vi "Initialize.vi"(8 "ErrorIn":errorcluster, 10 "Modul Type to Simulate":T1 items=["Hardware Modus"=0, "SPC-600 Simulation"=600, "SPC-630 Simulation"=630, "SPC-700  Simulation"=700, "SPC-730  Simulation"=730, "SPC-130  Simulation"=130, "SPC-830  Simulation"=830, "SPC-140  Simulation"=140, "SPC-930  Simulation"=930, "DPC-230  Simulation"=230, "SPC-150  Simulation"=150, "SPC-150 N  Simulation"=151, "SPC-150 NX  Simulation"=152, "SPC-130 EM  Simulation"=131, "SPC-130 EMN  Simulation"=132, "SPC-130 IN Simulation"=135, "SPC-130 INX Simulation"=136, "SPC-130 INXX Simulation"=137, "SPC-160  Simulation"=160, "SPC-160 X  Simulation"=161, "SPC-160 PCIE  Simulation"=162, "SPC-180 Simulation"=180, "SPC-181 Simulation"=181, "SPC-182 Simulation"=182, "SPC-185 Simulation"=185, "SPC-186 Simulation"=186, "SPC-187 Simulation"=187, "DPC-330  Simulation"=330, "DPC-590  Simulation"=590, "TDC-104 Simulation"=104, "TDC-004 Simulation"=4, "TDC-106 Simulation"=106]) -> (0 "ErrorOut":errorcluster, 1 "SerialNumbersArray":string[](array[string]), 2 "ModuleNoArray":i16[](array[numeric]), 3 "DLL Path":path, 5 "SPCModulesArray":T2[](array[typedef]) {"Bus Number" min=-1 max=255 step=1; "Base I/O Addr" format="%.0x"; "Init Status" min=-10 max=0 step=1; "in Use" min=-1 max=1 step=1; "Slot Number" min=-1 max=255 step=1; "Module Type" items=["SPC-600"=600, "SPC-630"=630, "SPC-700"=700, "SPC-730"=730, "SPC-130"=130, "SPC-830"=830, "SPC-140"=140, "SPC-930"=930, "DPC-230"=230, "SPC-150"=150, "SPC-150 N"=151, "SPC-150 NX"=152, "SPC-130 EM"=131, "SPC-130 EMN"=132, "SPC-130IN"=135, "SPC-130INX"=136, "SPC-130INXX"=137, "SPC-160"=160, "SPC-160 X"=161, "SPC-160 PCIE"=162, "SPC-180 N"=180, "SPC-180 NX"=181, "SPC-180 NXX"=182, "SPC-180 N-USB"=185, "SPC-180 NX-USB"=186, "SPC-180 NXX-USB"=187, "SPC-QC-104"=104, "SPC-QC-004"=4, "SPC-QC-106"=106, "DPC-330"=330, "PMS-800"=800, "SPC-590"=590, "Simulation"=-1]})   [LabVIEW 2023]
doc: "This is a convenience VI combining several spcmdll calls all needed to successfully initialize communication to SPC modules.\nBefore a measurement is started the measurement parameter values must be written into the internal structures of the DLL functions (not directly visible from the user program) and sent to the control registers of the SPC module(s). This is accomplished by the function SPC_init. The function\n- checks whether DLL is correctly registered ( looks for a BH license number and verifies it)\n- reads the parameter values from the specified file ini_file\n- checks and recalculates the parameters depending on hardware restrictions and adjust parameters from the EEPROM on the SPC module(s)\n- sends the parameter values to the internal structures of the DLL \n- sends the parameter values to the SPC control registers\n- performs a hardware test of the SPC module(s)\nThe module will be initialised, but only when it is not in use (locked) by other application.\nAfter successful initialisation the module is locked to prevent that other application can access it. The user should check initialisation status of all modules he wants to use by calling SPC_get_init_status function.\nIf, for some reasons, the module which was locked must be initialised, it can be done using the function SPC_set_mode with the parameter 'force_use' = 1. \nThe initialisation file is an ASCII file with a structure shown in the table below. We recommend either to use the file spcm.ini or to start with spcm.ini and introduce the desired changes.\n\ninfo@becker-hickl.com"
uses:
  SPC_Controls/SPCModInfo.ctl
  SPC_Controls/ModuleType.ctl
  SPC_Controls/ModuleTypes.ctl
panel:
  out "Number of Usable Modules":i16 min=0 max=8
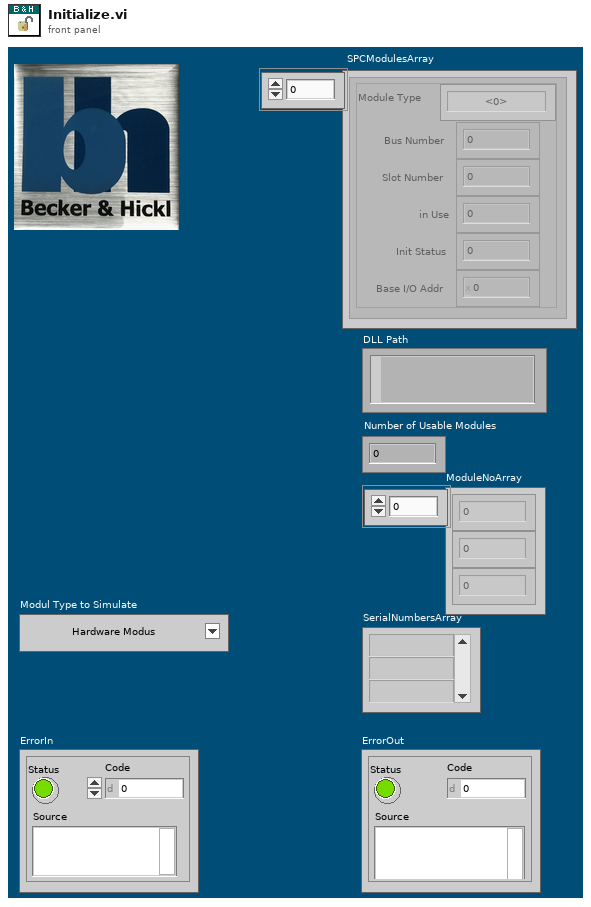
[diagram p1: front panel]
types:
  T1 = typedef "ModuleTypes.ctl" = i16
  T2 = typedef "SPCModInfo.ctl" = cluster{"Module Type":T3, "Bus Number":i16, "Slot Number":i16, "in Use":i16, "Init Status":i16, "Base I/O Addr":u16}
  T3 = typedef "ModuleType.ctl" = i16
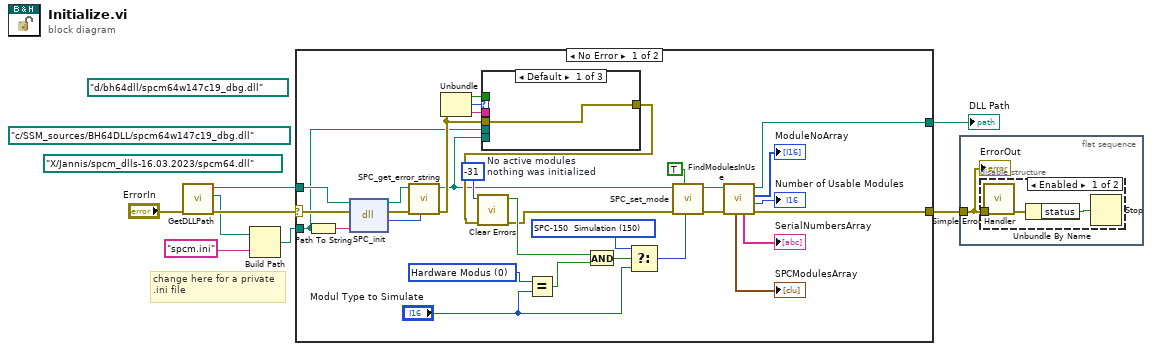
[diagram p0: block diagram]
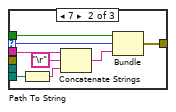
[diagram p3: hidden frame]
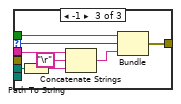
[diagram p4: hidden frame]
diagram:
  (unwired) path "X:/Jannis/spcm_dlls-16.03.2023/spcm64.dll" ("DLL Path")
  (unwired) path "c:/SSM_sources/BH64DLL/spcm64w147c19_dbg.dll" ("DLL Path")
  (unwired) path "d:/bh64dll/spcm64w147c19_dbg.dll" ("DLL Path")
  # "change here for a private\n.ini file"
  n1 = call "GetDLLPath.vi"("Error In"="ErrorIn") -> ("Error Out"=w7:errorcluster, "SPC Folder Path"=w2:path, "DLL Path"=w1:path)  [unwired: 7 in, 1 out]
  n2 = Build Path(base path=w2, name or relative path="spcm.ini") -> (appended path=w4:path)
  n3 = case shown="No Error" w7 {
    selector: w7 -> [w27 w58]
    tunnel: [w39 w57] -> w6
    tunnel: w1 -> [w26 w57]
    tunnel: [w38 w58] -> w5
    tunnel: w4 -> [w12 _]
    frame No Error {
      w19 = T1 0 items=["Hardware Modus"=0, "SPC-600 Simulation"=600, "SPC-630 Simulation"=630, "SPC-700  Simulation"=700, "SPC-730  Simulation"=730, "SPC-130  Simulation"=130, "SPC-830  Simulation"=830, "SPC-140  Simulation"=140, "SPC-930  Simulation"=930, "DPC-230  Simulation"=230, "SPC-150  Simulation"=150, "SPC-150 N  Simulation"=151, "SPC-150 NX  Simulation"=152, "SPC-130 EM  Simulation"=131, "SPC-130 EMN  Simulation"=132, "SPC-160  Simulation"=160, "SPC-160 X  Simulation"=161, "SPC-160 PCIE  Simulation"=162, "DPC-330  Simulation"=330, "DPC 590  Simulation"=590] ("x")
      w23 = T1 150 items=["Hardware Modus"=0, "SPC-600 Simulation"=600, "SPC-630 Simulation"=630, "SPC-700  Simulation"=700, "SPC-730  Simulation"=730, "SPC-130  Simulation"=130, "SPC-830  Simulation"=830, "SPC-140  Simulation"=140, "SPC-930  Simulation"=930, "DPC-230  Simulation"=230, "SPC-150  Simulation"=150, "SPC-150 N  Simulation"=151, "SPC-150 NX  Simulation"=152, "SPC-130 EM  Simulation"=131, "SPC-130 EMN  Simulation"=132, "SPC-160  Simulation"=160, "SPC-160 X  Simulation"=161, "SPC-160 PCIE  Simulation"=162, "DPC-330  Simulation"=330, "DPC 590  Simulation"=590] ("t")
      w24 = -31  # No active modules nothing was initialized
      n4 = Path To String(path=w12) -> (string=w28:string)
      n5 = dll-call lib="D:/spcm/lib/lab_view/lv10.0/spcm32.dll" fn="SPC_init"(path in=w26, error in=w27, "ini_file"=w28) -> (path out=w29:path, error out=w31:errorcluster, "return type"=w30:i16)  [unwired: 2 in]
      n6 = call "SPC_get_error_string.vi"("ErrorID"=w30, "Error In"=w31, "DLL Path"=w29) -> ("Error Out"=w13:errorcluster, "DLL Path"=w11:path)  [unwired: 6 in, 1 out]
      n7 = Unbundle(w13) -> ("Status"=w15:bool, "Code"=w17:i32, "Source"=w16:string)
      n8 = case shown="Default" w17 {
        selector: w17 -> [_ w43 w52]
        tunnel: w16 -> [_ w48 w56]
        tunnel: w11 -> [_ w47 _]
        tunnel: w15 -> [_ w42 w51]
        tunnel: [w40 w41 w50] -> w14
        tunnel: w13 -> [w40 _ _]
        tunnel: w12 -> [_ _ w49]
        frame Default {
        }
        frame 7 {
          n9 = Path To String(path=w47) -> (string=w46:string)
          n10 = Concatenate Strings(w48, "\r", w46) -> (w44:string)
          n11 = Bundle("Status"=w42, "Code"=w43, w44) -> (w41:cluster{"Status":bool, "Code":i32, string})  [unwired: 1 in]
        }
        frame -1 {
          n12 = Path To String(path=w49) -> (string=w55:string)
          n13 = Concatenate Strings(w56, "\r", w55) -> (w53:string)
          n14 = Bundle("Status"=w51, "Code"=w52, w53) -> (w50:cluster{"Status":bool, "Code":i32, string})  [unwired: 1 in]
        }
      }
      n15 = call <vilib>:"Clear Errors.vi"("error in (no error)"=w14, "specific error code to clear (0: all)"=w24) -> ("error out"=w9:errorcluster, "specific error cleared?"=w22:bool)  [unwired: 4 in]
      n16 = Equal?(x=w19, y="Modul Type to Simulate") -> (x = y?=w18:bool)
      n17 = And(x=w22, y=w18) -> (x .and. y?=w21:bool)
      n18 = Select(t=w23, s=w21, f="Modul Type to Simulate") -> (s? t:f=w25:T1)
      n19 = call "SPC_set_mode.vi"("Modul Type to Simulate"=w25, "Force Use"=TRUE, "Error In"=w9, "DLL Path"=w11) -> ("Error Out"=w32:errorcluster, "DLL Path"=w33:path)  [unwired: 6 in]
      n20 = call "FindModulesInUse.vi"("Error In"=w32, "DLL Path"=w33) -> ("Error Out"=w38:errorcluster, "Number of Usable Modules"=→"Number of Usable Modules":i16, "ModuleNoArray"=→"ModuleNoArray":i16[], "DLL Path"=w39:path, "Array Of Serialnumbers"=→"SerialNumbersArray":string[], "SPCModulesArray"=→"SPCModulesArray":T2[])  [unwired: 4 in]
    }
    frame Error {
    }
  }
  "DLL Path" <- w6
  n21 = flat-sequence {
    tunnel: w5 -> [w59]
    frame #0 {
      n22 = disable-structure shown="Enabled" {
        disable-tunnel: w59 -> [w61 _]
        frame Enabled {
          n23 = call <vilib>:"Simple Error Handler.vi"("error in (no error)"=w61) -> ("error out"=w60:errorcluster)  [unwired: 4 in, 4 out]
          n24 = Unbundle By Name(w60) -> ("status"=w62:bool)
          n25 = Stop(stop? (T)=w62) -> ()
        }
        frame Disabled {
        }
      }
      "ErrorOut" <- w59
    }
  }
